vi "RichToFlatsift_proxy_v1_CreateLabviewIngestionConfigResponse.vi"(5 "OutputClusterType":T1, 11 "InputCluster":T2) -> (3 "OutputCluster":T1)   [LabVIEW 2024, in "SiftProxy_client.lvlib"]
uses:
  sift_proxy_v1_CreateLabviewIngestionConfigResponse.ctl
  sift_proxy_v1_CreateLabviewIngestionConfigResponse_Flat.ctl
  SiftProxy_client.lvlib
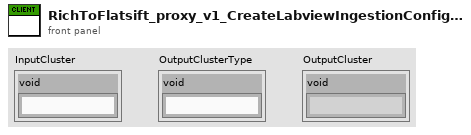
[diagram p1: front panel]
types:
  T1 = typedef "SiftProxy_client.lvlib/sift_proxy_v1_CreateLabviewIngestionConfigResponse_Flat.ctl" = cluster{"void":string}
  T2 = typedef "SiftProxy_client.lvlib/sift_proxy_v1_CreateLabviewIngestionConfigResponse.ctl" = cluster{"void":string}
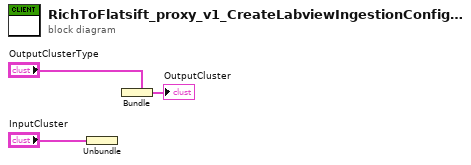
[diagram p0: block diagram]
diagram:
  n1 = Unbundle "Unbundle"("InputCluster") -> ()  [unwired: 1 out]
  n2 = Bundle "Bundle"(cluster="OutputClusterType") -> (→"OutputCluster":T1)  [unwired: 1 in]
